vi "While Loop Subdiagram Label.vi"(6 "Variant in":variant, 7 "Shift Pressed?":bool, 8 "error in (no error)":errorcluster, 10 "QD Combo Box Ref":refnum<vi>, 11 "QD Launch VI Ref":refnum<vi>) -> (0 "error out":errorcluster, 4 "Variant out":variant)   [LabVIEW 2020, in "While Loop Subdiagram Label.lvlib"]
doc: "Takes the text in the Quick Drop box and applies it as a subdiagram label to a While Loop, and formats the subdiagram label to have white, bold text, with the while loop's gray background color."
uses:
  While Loop Subdiagram Label.lvlib
panel:
  in  "Undo Name":string="While Loop Subdiagram Label"
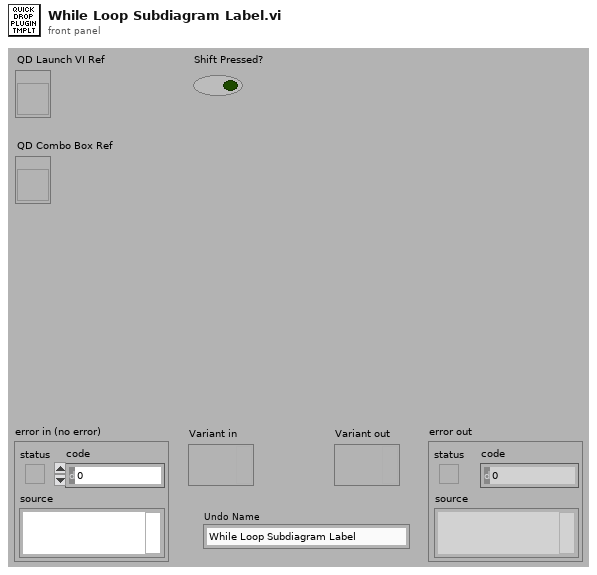
[diagram p1: front panel]
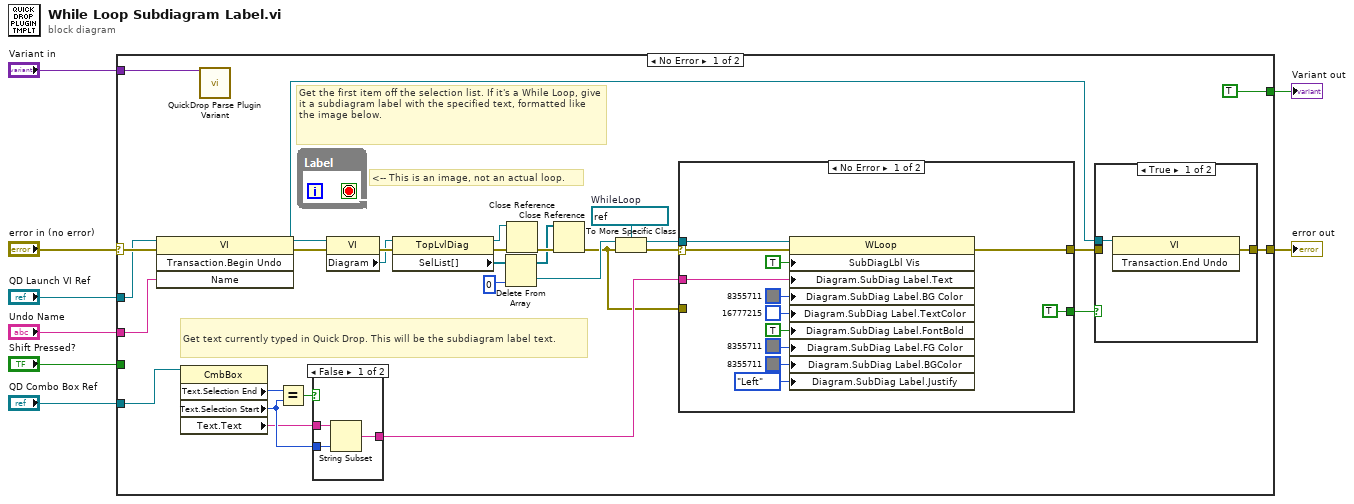
[diagram p0: block diagram]
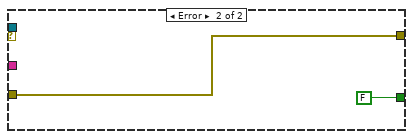
[diagram p2: hidden frame]
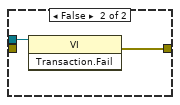
[diagram p4: hidden frame]
diagram:
  n1 = case shown="No Error" "error in (no error)" {
    selector: "error in (no error)" -> [w36 w60]
    tunnel: [w31 w60] -> w7
    tunnel: "QD Launch VI Ref" -> [w35 _]
    tunnel: "Shift Pressed?" -> [_ _]
    tunnel: "QD Combo Box Ref" -> [w20 _]
    tunnel: "Variant in" -> [w37 _]
    tunnel: "Undo Name" -> [w34 _]
    tunnel: [TRUE _] -> w1
    frame No Error {
      w15 = refnum<vi> refnum  # WhileLoop
      # "Get text currently typed in Quick Drop. This will be the subdiagram label text."
      # "<-- This is an image, not an actual loop."
      # "Get the first item off the selection list. If it's a While Loop, give it a subdiagram label with the specified text, formatted like the image below."
      n2 = invoke class="VI" method="Transaction.Begin Undo"(reference=w35, error in=w36, "Name"=w34) -> (reference out=w29:refnum<vi>, error out=w32:errorcluster)  [unwired: 1 in, 2 out]
      n3 = property on="Property Node" class="CmbBox"(reference=w20) -> ("Text.Selection End"=w24:u32, "Text.Selection Start"=w22:u32, "Text.Text"=w21:string)  [unwired: 1 in, 2 out]
      n4 = call <vilib>:"QuickDrop Parse Plugin Variant.vi"("QDKS Variant in"=w37) -> ()  [unwired: 12 in, 3 out]
      n5 = Equal?(x=w24, y=w22) -> (x = y?=w23:bool)
      n6 = case shown="False" w23 {
        tunnel: [w54 w55] -> w11
        tunnel: w22 -> [w53 _]
        tunnel: w21 -> [w52 w55]
        frame False {
          n7 = String Subset(string=w52, length (rest)=w53) -> (substring=w54:string)  [unwired: 1 out]
        }
        frame True {
        }
      }
      n8 = property class="VI"(reference=w29, error in=w32) -> (error out=w28:errorcluster, "Diagram"=w27:refnum<vi>)  [unwired: 1 out]
      n9 = property class="TopLvlDiag"(reference=w27, error in=w28) -> (reference out=w25:refnum<vi>, error out=w26:errorcluster, "SelList[]"=w18:refnum<vi>[])
      n10 = Delete From Array(array=w18, index=0) -> (deleted portion=w16:refnum<vi>, array with subset deleted=w17:refnum<vi>[])  [unwired: 1 in]
      n11 = Close Reference(reference=w25, error in (no error)=w26) -> (error out=w30:errorcluster)
      n12 = Close Reference(reference=w17, error in (no error)=w30) -> (error out=w9:errorcluster)
      n13 = To More Specific Class(target class=w15, reference=w16, error in=w9) -> (specific class reference=w12:refnum<vi>, error out=w14:errorcluster)
      n14 = case shown="No Error" w14 {
        selector: w14 -> [w48 _]
        tunnel: [TRUE FALSE] -> w13
        tunnel: w12 -> [w47 _]
        tunnel: w11 -> [w46 _]
        tunnel: [w43 w50] -> w10
        tunnel: w9 -> [_ w50]
        frame No Error {
          n15 = property class="WLoop"(reference=w47, error in=w48, "SubDiagLbl Vis"=TRUE ("Subdiagram Label Visible"), "Diagram.SubDiag Label.Text"=w46, "Diagram.SubDiag Label.BG Color"=u32 8355711, "Diagram.SubDiag Label.TextColor"=u32 16777215, "Diagram.SubDiag Label.FontBold"=TRUE ("Diagram.Subdiagram Label.Font:Bold"), "Diagram.SubDiag Label.FG Color"=u32 8355711, "Diagram.SubDiag Label.BGColor"=u32 8355711, "Diagram.SubDiag Label.Justify"=enum16{"Left", "Center", "Right"}."Left" ("Diagram.Subdiagram Label.Justification")) -> (error out=w43:errorcluster)  [unwired: 1 out]
        }
        frame Error {
        }
      }
      n16 = case shown="True" w13 {
        tunnel: w29 -> [w56 w58]
        tunnel: [w57 w59] -> w31
        tunnel: w10 -> [_ _]
        frame True {
          n17 = invoke class="VI" method="Transaction.End Undo"(reference=w56) -> (error out=w57:errorcluster)  [unwired: 2 in, 2 out]
        }
        frame False {
          n18 = invoke class="VI" method="Transaction.Fail"(reference=w58) -> (error out=w59:errorcluster)  [unwired: 2 in, 2 out]
        }
      }
    }
    frame Error {
    }
  }
  "error out" <- w7
  "Variant out" <- w1
